vi "driveHold.vi"(11 "time":dbl) -> ()   [LabVIEW 2011]
uses:
  common/scale_const.ctl
  drivetrain/gear_shift_state.ctl
  drivetrain/drivetrain_drive_mode.ctl
  drivetrain/drivetrain_drive_write_thread.ctl
  drivetrain/drivetrain_globals.vi
panel:
  in  "forward bias":dbl
  out "x+y":u32
  out "unsigned 32bit integer":u32
  in  "Scale Const":T1={"min_ana"=0.0, "min_units"=6.0, "max_ana"=24.0, "max_units"=0.0}
  in  "absolute integral cap":dbl=6.0
  in  "kI":dbl=-0.005
  out "x > y?":bool
  out "Waveform Chart":cluster{"Left":dbl, "Right":dbl}(graph)
  in  "max hold speed":dbl=8.0
  in  "kP":dbl=-0.5
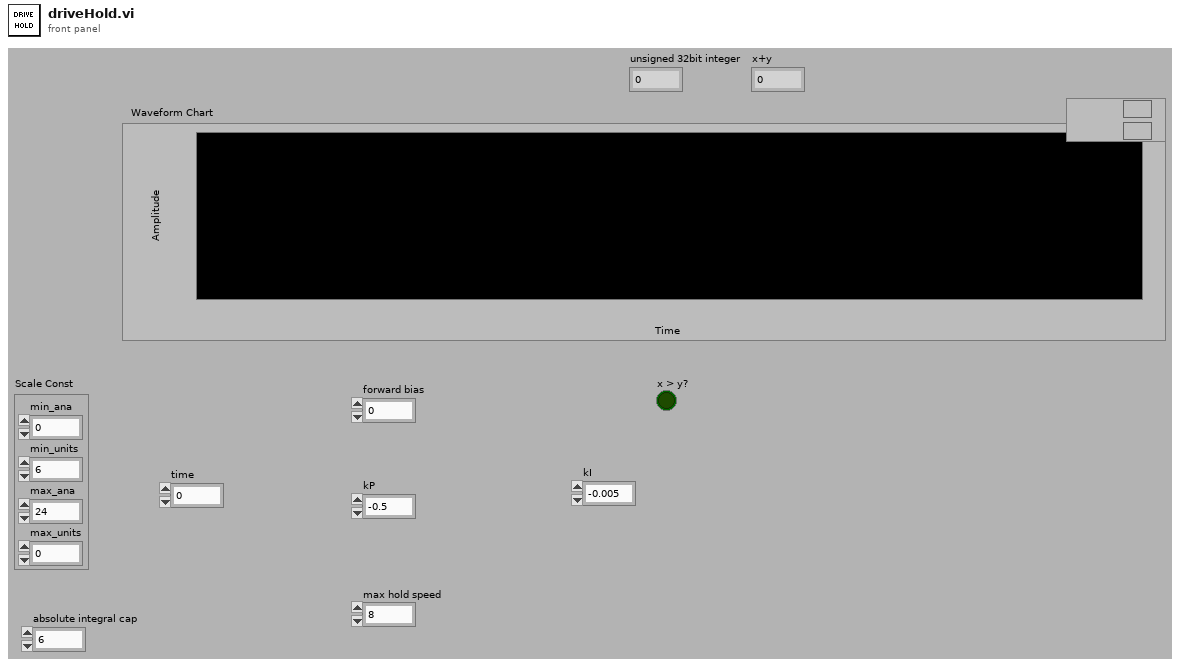
[diagram p1: front panel]
types:
  T1 = typedef "scale_const.ctl" = cluster{"min_ana":dbl, "min_units":dbl, "max_ana":dbl, "max_units":dbl}
  T2 = typedef "gear_shift_state.ctl" = enum16{"low", "high"}
  T3 = typedef "drivetrain_drive_mode.ctl" = enum16{"open loop", "closed loop"}
  T4 = typedef "drivetrain_drive_write_thread.ctl" = enum16{"Teleop", "Script Engine - Autonomous", "Script Engine - Sequence"}
  T5 = typedef "WPI_RobotDriveDevRef.ctl" = cluster{"DevStatus":errorcluster, "Motors[]":T6[], "Square Inputs":bool, "Max Output":dbl}
  T6 = typedef "WPI_MotorControlDeviceRef.ctl" = cluster{"DeviceStatus":errorcluster, "Type":enum16{"PWM", "CAN"}, "PWM":cluster{"Digital Module":T7, "PWM Channel":T8, "DeadBand":T9}, "CAN":cluster{"Device Number":u8, "Control Mode":T10, "Semaphore":T11, "Max Vout":dbl}, "Invert":bool, "TransformRef":T12, "InvTransformRef":T12}
  T7 = typedef "FPGA_TypedefDigitalModule.ctl" = enum16{"Digital Module 1", "Digital Module 2"}
  T8 = typedef "FPGA_DIOPWMChannel.ctl" = enum8{"PWM 1", "PWM 2", "PWM 3", "PWM 4", "PWM 5", "PWM 6", "PWM 7", "PWM 8", "PWM 9", "PWM 10", "Invalid"}
  T9 = typedef "WPI_PWMDeadband.ctl" = cluster{"Name":string, "maxPositivePwm":i32, "minPositivePwm":i32, "centerPwm":i32, "maxNegativePwm":i32, "minNegativePwm":i32, "angularRange":u16}
  T10 = typedef "WPI_CANJaguar_ControlMode.ctl" = enum8{"Percent VBus", "Current", "Speed", "Position", "Voltage"}
  T11 = typedef "Semaphore RefNum" = refnum<k1>
  T12 = typedef "WPI_PWMTransform_ConPane.ctl" = refnum<vi>
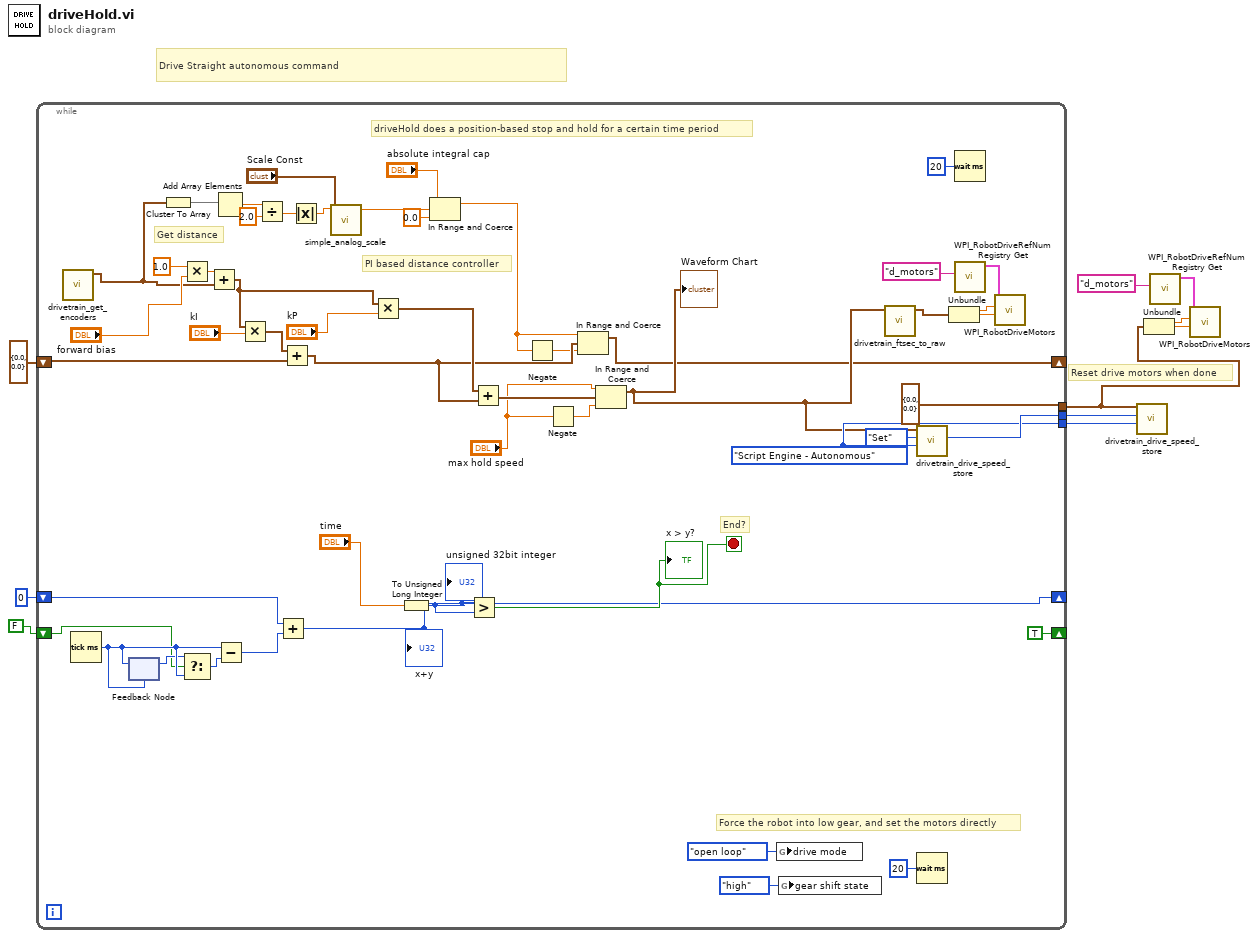
[diagram p0: block diagram]
diagram:
  # "Drive Straight autonomous command"
  # "Reset drive motors when done"
  n1 = while {
    tunnel: [cluster{"Left":dbl, "Right":dbl} {"Left"=0.0, "Right"=0.0} ("Drive")] -> w6
    tunnel: [w58] -> w10
    tunnel: [w57] -> w9
    shift-right: [w35] -> _
    shift-left: cluster{"Left":dbl, "Right":dbl} {"Left"=0.0, "Right"=0.0} -> [w48]
    shift-right: [w39] -> _
    shift-left: u32 0 -> [w42]
    shift-right: [TRUE] -> _
    shift-left: FALSE -> [w17]
    stop <- w40 stop-if-true
    w57 = drivetrain_drive_write_thread."Script Engine - Autonomous" ("Write Thread")
    w58 = enum16{"Set", "Get"}."Set" ("data_store_mode")
    # "driveHold does a position-based stop and hold for a certain time period"
    # "PI based distance controller"
    # "Get distance"
    # "End?"
    # "Force the robot into low gear, and set the motors directly"
    n2 = call "drivetrain_get_encoders.vi"() -> ("Distance (in)"=w11:cluster{"Left":dbl, "Right":dbl})  [unwired: 9 in, 2 out]
    n3 = Tick Count (ms)() -> (millisecond timer value=w20:u32)
    n4 = feedback-in #1(w20) -> ()
    n5 = feedback #1(w20) -> (w18:u32)
    n6 = Cluster To Array(cluster=w11) -> (array=w34:dbl[])
    n7 = Multiply(x=1.0, y="forward bias") -> (x*y=w14:dbl)
    n8 = Select(t=w18, s=w17, f=w20) -> (s? t:f=w19:u32)
    n9 = Add(x=w14, y=w11) -> (x+y=w15:cluster{"Left":dbl, "Right":dbl})
    n10 = Add Array Elements(numeric array=w34) -> (sum=w33:dbl)
    n11 = Subtract(x=w20, y=w19) -> (x-y=w41:u32)
    n12 = Multiply(x=w15, y="kI") -> (x*y=w37:cluster{"Left":dbl, "Right":dbl})
    n13 = Divide(x=w33, y=2.0) -> (x/y=w22:dbl)
    n14 = Add(x=w42, y=w41) -> (x+y=w39:u32)
    "x+y" <- w39
    n15 = Add(x=w37, y=w48) -> (x+y=w36:cluster{"Left":dbl, "Right":dbl})
    n16 = Absolute Value(x=w22) -> (abs(x)=w21:dbl)
    n17 = call "simple_analog_scale.vi"("Scale Const"="Scale Const", "Analog"=w21) -> ("Units"=w31:dbl)  [unwired: 9 in]
    n18 = Multiply(x=w15, y="kP") -> (x*y=w47:cluster{"Left":dbl, "Right":dbl})
    n19 = To Unsigned Long Integer(number="time") -> (unsigned 32bit integer=w25:u32)
    "unsigned 32bit integer" <- w25
    n20 = In Range and Coerce(upper limit="absolute integral cap", x=w31, lower limit=0.0) -> (coerced(x)=w29:dbl)  [unwired: 1 out]
    n21 = Greater?(x=w39, y=w25) -> (0:w40:bool)
    "x > y?" <- w40
    n22 = Add(x=w47, y=w36) -> (x+y=w46:cluster{"Left":dbl, "Right":dbl})
    n23 = Negate(x=w29) -> (-x=w30:dbl)
    n24 = Negate(x="max hold speed") -> (-x=w45:dbl)
    n25 = In Range and Coerce(upper limit=w29, x=w36, lower limit=w30) -> (coerced(x)=w35:cluster{"Left":dbl, "Right":dbl})  [unwired: 1 out]
    n26 = In Range and Coerce(upper limit="max hold speed", x=w46, lower limit=w45) -> (coerced(x)=w43:cluster{"Left":dbl, "Right":dbl})  [unwired: 1 out]
    "Waveform Chart" <- w43
    n27 = global write "drivetrain_globals.vi" "drive mode"(drivetrain_drive_mode."open loop" ("drive mode")) -> ()
    n28 = global write "drivetrain_globals.vi" "gear shift state"(gear_shift_state."high" ("gear shift state")) -> ()
    n29 = call "drivetrain_ftsec_to_raw.vi"("Drive Data"=w43) -> ("Drive Data Out"=w50:cluster{"Left":dbl, "Right":dbl})  [unwired: 10 in]
    n30 = call "drivetrain_drive_speed_store.vi"("Write Thread"=w57, "data_store_mode"=w58, "drive data"=w43) -> ()  [unwired: 7 in, 2 out]
    n31 = Wait (ms)(milliseconds to wait=u32 20) -> ()  [unwired: 1 out]
    n32 = Unbundle(w50) -> ("Left"=w52:dbl, "Right"=w53:dbl)
    n33 = Wait (ms)(milliseconds to wait=u32 20) -> ()  [unwired: 1 out]
    n34 = call <vilib>:"WPI_RobotDriveRefNum Registry Get.vi"("refnum name"="d_motors") -> ("RobotDriveDevRef"=w55:T5)  [unwired: 9 in, 1 out]
    n35 = call <vilib>:"WPI_RobotDriveMotors.vi"("RightSpeed"=w53, "LeftSpeed"=w52, "RobotDriveDevRef"=w55) -> ()  [unwired: 7 in, 2 out]
  }
  n36 = call "drivetrain_drive_speed_store.vi"("Write Thread"=w9, "data_store_mode"=w10, "drive data"=w6) -> ()  [unwired: 7 in, 2 out]
  n37 = Unbundle(w6) -> ("Left"=w8:dbl, "Right"=w7:dbl)
  n38 = call <vilib>:"WPI_RobotDriveRefNum Registry Get.vi"("refnum name"="d_motors") -> ("RobotDriveDevRef"=w4:T5)  [unwired: 9 in, 1 out]
  n39 = call <vilib>:"WPI_RobotDriveMotors.vi"("RightSpeed"=w7, "LeftSpeed"=w8, "RobotDriveDevRef"=w4) -> ()  [unwired: 7 in, 2 out]
